vi "Actor Core_Temp.vi"() -> ()   [LabVIEW 2023, in "SLM_Controller.lvlib" / "SLM_Controller.lvclass"]
uses:
  SLM_Controller.lvclass
  SLM_Controller.lvclass/SLM_Controller.ctl
panel:
  out "Background Zero Array":i8[][](array[numeric])
  out "Background  Graph":sgl[][](graph)
  out "Background Phases":dbl[][][](array[numeric])
  out "Aperture Mask":sgl[][](array[numeric])
  out "Python session 2":refnum<k35>
  out "Python session 1":refnum<k35>
  out "SLM Max Width":i32
  out "SLM Max Height":i32
  out "slm error out 2":errorcluster
  out "Zero array":i8[][](array[numeric])
  out "Control File Path":path
  out "Phases":dbl[][][](array[numeric])
  in  "SLM Width":i32=600
  in  "SLM Height":i32=600
  out "Current Phases":sgl[][](graph)
  in  "SLM Phases":T1(tab)
  in  "Grating Sliders":T2 {"Y" scale=0.0..50.0; "X" scale=0.0..50.0}
  in  "SuperPixel Y":i8=1 min=1
  in  "SuperPixel X":i8=1 min=1
  in  "SuperPixel Array":sgl[][](array[numeric]) min=0 max=2 format="%#_3g"
  in  "SuperPixelArray_On_Off":bool
  in  "Checkerboard":T3={"Multiplier A"=0.0, "Multiplier B"=0.0, "Super Pixel Y"=1, "Super Pixel X"=1} {"Super Pixel X" min=1; "Super Pixel Y" min=1; "Multiplier B" scale=0.0..2.0; "Multiplier A" scale=0.0..2.0}
  in  "Phase Array Checkerboard":bool
  in  "Fresnel_On_Off":bool
  in  "Fresnel Lens":T4={"Wavelength"=1, "Focal Length"=1.0, "N"=0.0, "x_0"=0.0, "y_0"=0.0} {"y_0" scale=0.0..100.0; "x_0" scale=0.0..100.0; "N" scale=1.0..10.0; "Focal Length" min=1.0 max=500.0 scale=1.0..2000.0; "Wavelength" min=1 scale=1.0..1000.0}
  in  "Vortex Checkerboard On/Off":bool
  in  "Vortex_On_Off":bool
  in  "Vortex Checkerboard":T5={"Topological Charge A"=0, "Topological Charge B"=0, "VortexPixel Y"=1, "VortexPixel X"=1} {"VortexPixel X" min=1; "VortexPixel Y" min=1; "Topological Charge B" scale=-10.0..10.0; "Topological Charge A" scale=-10.0..10.0}
  in  "VortexPixel X":i8=1 min=1
  in  "VortexPixel Y":i8=1 min=1
  in  "Vortex Array":dbl[][](array[numeric])
  in  "Laguerre_On_Off":bool
  in  "Laguerre_Gaussian":T6={"L"=1, "P"=0, "w_0"=1, "x_0"=0.0, "y_0"=0.0} {"y_0" scale=0.0..100.0; "x_0" scale=0.0..100.0; "w_0" min=1 max=500 scale=1.0..500.0; "P" min=0 step=1 scale=0.0..10.0; "L" min=1 scale=1.0..10.0}
  in  "Hermite Gaussian":T7={"n"=1, "m"=0, "w_0"=1.0, "x_0"=0.0, "y_0"=0.0} {"y_0" scale=0.0..100.0; "x_0" scale=0.0..100.0; "w_0" min=1.0 max=500.0 scale=1.0..500.0; "m" min=0 step=1 scale=0.0..10.0; "n" min=1 scale=1.0..10.0}
  in  "Hermite_On_Off":bool
  in  "Axicon_On_Off":bool
  in  "Axicon Settings":cluster{"r_0":dbl, "x_0":dbl, "y_0":dbl}={"r_0"=1.0, "x_0"=0.0, "y_0"=0.0} {"y_0" scale=0.0..100.0; "x_0" scale=0.0..100.0; "r_0" min=1.0 scale=1.0..100.0}
  in  "Bessel_On_Off":bool
  in  "Bessel Settings":T8={"Topological Charge"=1, "Wavelength"=1, "Refractive Index"=0.0, "Degree"=0.0} {"Degree" scale=0.0..2.0; "Refractive Index" scale=0.0..2.0; "Wavelength" min=1 scale=1.0..1000.0; "Topological Charge" min=1 scale=1.0..10.0}
  in  "Airy_On_Off":bool
  in  "Airy Settings":cluster{"Power":i8, "Denominator":i8} {"Denominator" scale=1.0..10.0; "Power" scale=0.0..10.0}
  in  "Options Tap":enum32{"Aperture", "Background"}(tab)
  in  "Aperture Array":i16[][](array[numeric]) min=1
  in  "Aperture Pixel Y":i8=1 min=1
  in  "Aperture Pixel X":i8=1 min=1
  in  "Aperture Checkerboard":T9={"Multiplier A"=1, "Multiplier B"=1, "Aperture Pixel Y"=1, "Aperture Pixel X"=1} {"Aperture Pixel X" min=1; "Aperture Pixel Y" min=1; "Multiplier B" min=1 scale=1.0..500.0; "Multiplier A" min=1 scale=1.0..800.0}
  in  "Aperture Checkerboard On/Off":bool
  in  "Background_Axicon_On_Off":bool
  in  "Background_Grating_On_Off":bool
  in  "Background_Fresnel_On_Off":bool
  in  "Fresnel":T4={"Wavelength"=1, "Focal Length"=1.0, "N"=0.0, "x_0"=0.0, "y_0"=0.0} {"Focal Length" min=1.0 max=500.0; "Wavelength" min=1}
  in  "Grating":T2
  in  "Axicon":cluster{"r_0":dbl, "x_0":dbl, "y_0":dbl}={"r_0"=1.0, "x_0"=0.0, "y_0"=0.0} {"r_0" min=1.0}
  out "Final Phase":dbl[][](graph)
  out "phases error out":errorcluster
  in  "Modulation Depth":dbl=214.0
  in  "SLM Monitor":i32=2
  in  "Correction Pattern":path=path "C:/Users/quantum/Desktop/SLM_SImple_GUI/correction_pattern_13138/CAL_LSH0802650_810nm.bmp"
  in  "Initialize SLM":bool
  in  "Continuous Button":bool
  in  "Single Upload":bool
  in  "Start/Stop":bool
  # "X"
  # "Y"
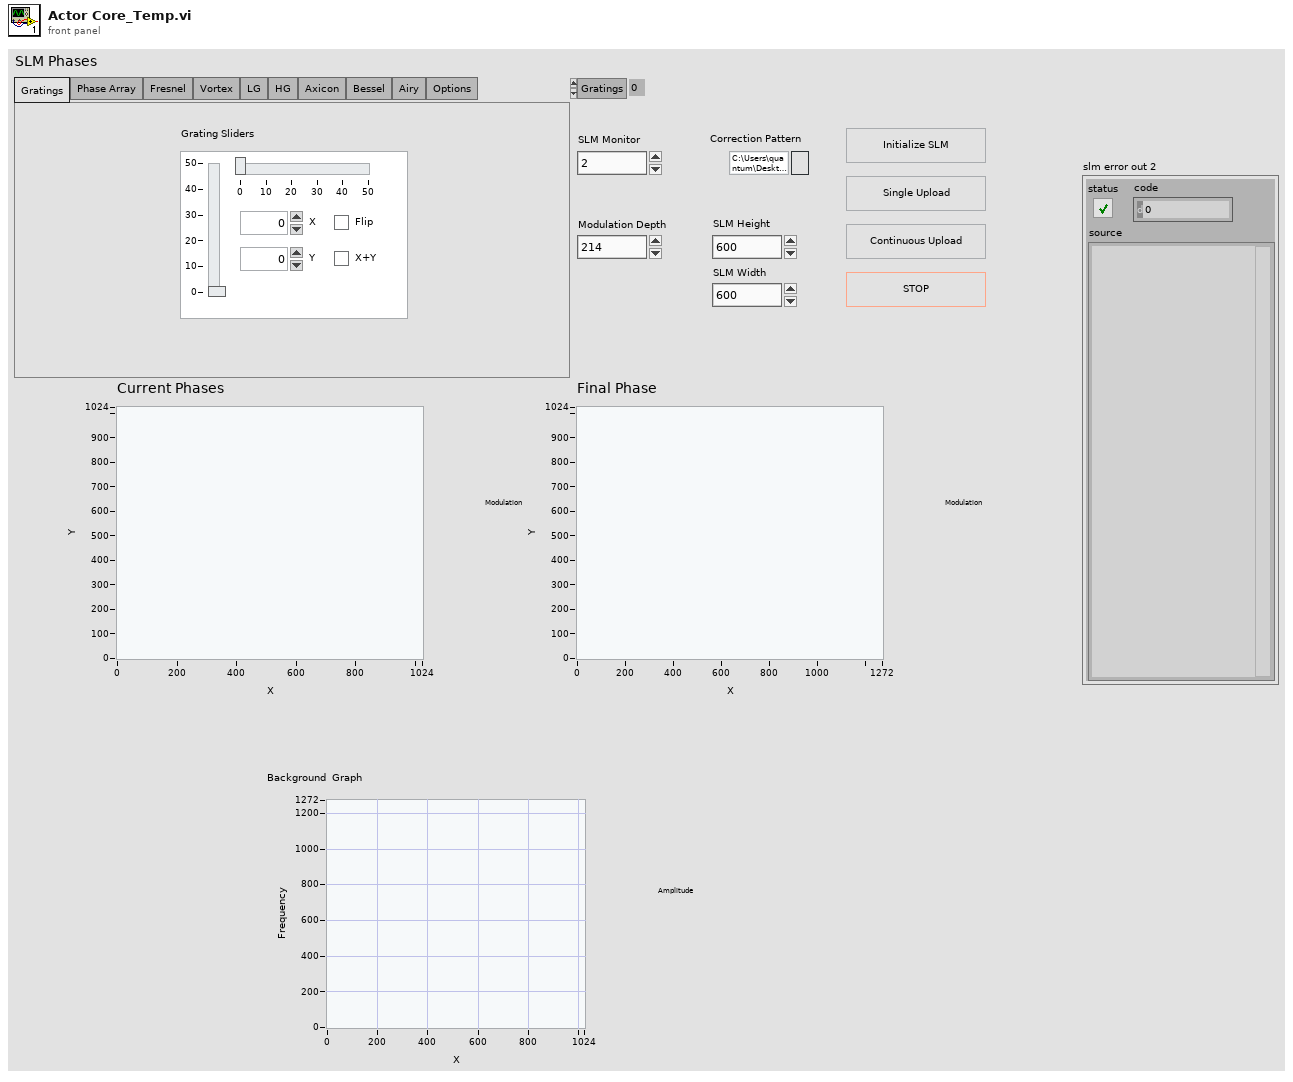
[diagram p1: front panel]
types:
  T1 = enum32{"Gratings", "Phase Array", "Fresnel", "Vortex", "LG", "HG", "Axicon", "Bessel", "Airy", "Options"}
  T2 = cluster{"X":i16, "Y":i16, "Flip":bool, "Orientation":bool}
  T3 = cluster{"Multiplier A":sgl, "Multiplier B":sgl, "Super Pixel Y":i8, "Super Pixel X":i8}
  T4 = cluster{"Wavelength":i16, "Focal Length":dbl, "N":dbl, "x_0":dbl, "y_0":dbl}
  T5 = cluster{"Topological Charge A":i8, "Topological Charge B":i8, "VortexPixel Y":i8, "VortexPixel X":i8}
  T6 = cluster{"L":i8, "P":i8, "w_0":i16, "x_0":dbl, "y_0":dbl}
  T7 = cluster{"n":i8, "m":i8, "w_0":dbl, "x_0":dbl, "y_0":dbl}
  T8 = cluster{"Topological Charge":i8, "Wavelength":i16, "Refractive Index":sgl, "Degree":sgl}
  T9 = cluster{"Multiplier A":i16, "Multiplier B":i16, "Aperture Pixel Y":i8, "Aperture Pixel X":i8}
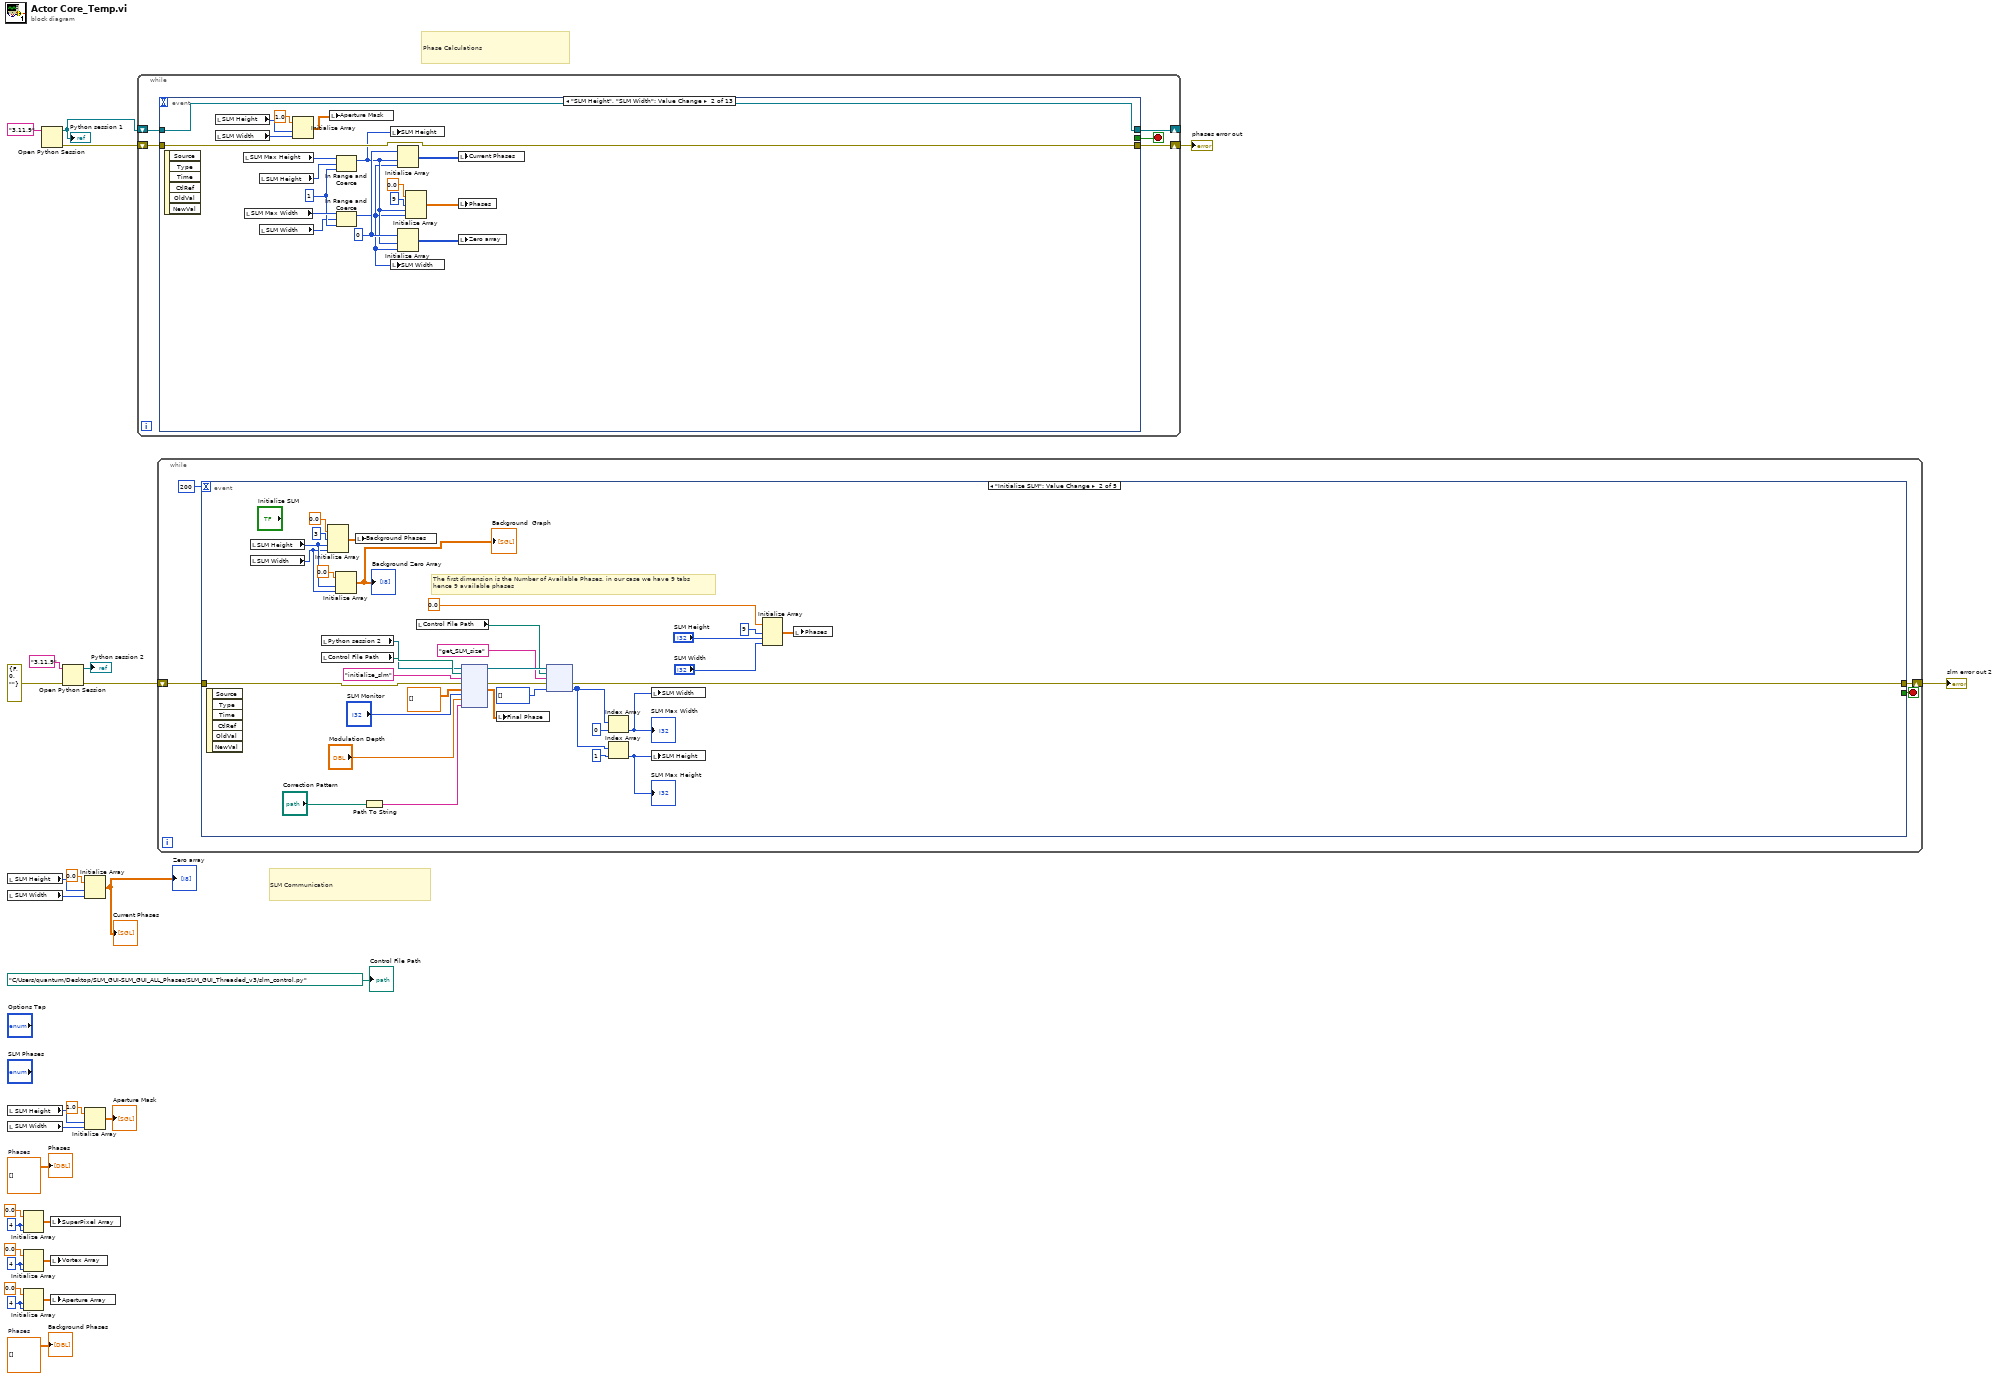
[diagram p0: block diagram]
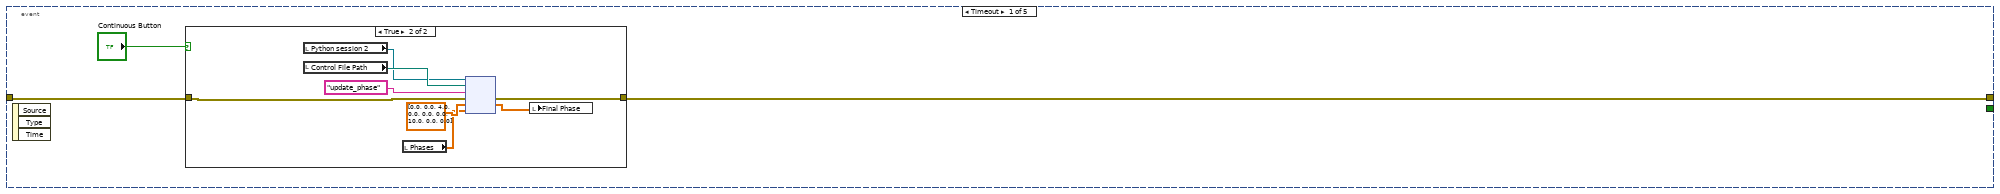
[diagram p2: hidden frame]
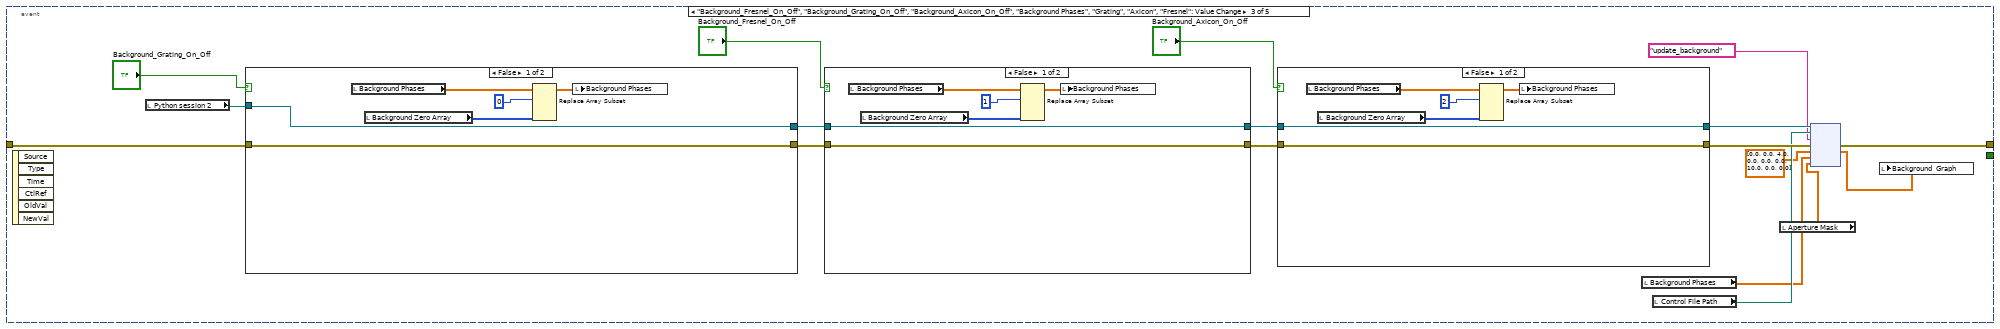
[diagram p4: hidden frame]
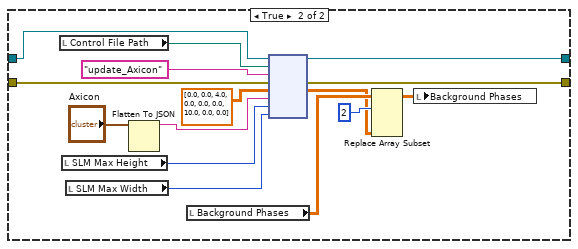
[diagram p5: hidden frame]
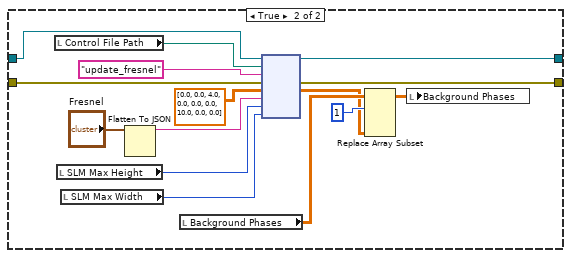
[diagram p6: hidden frame]
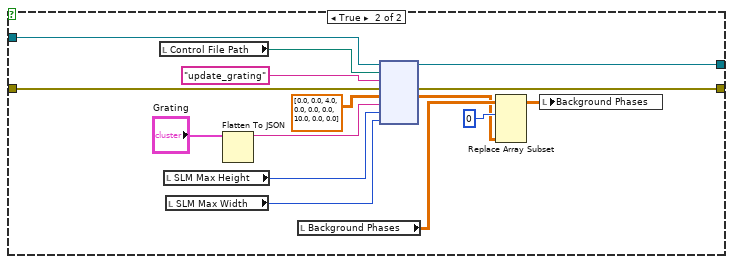
[diagram p7: hidden frame]
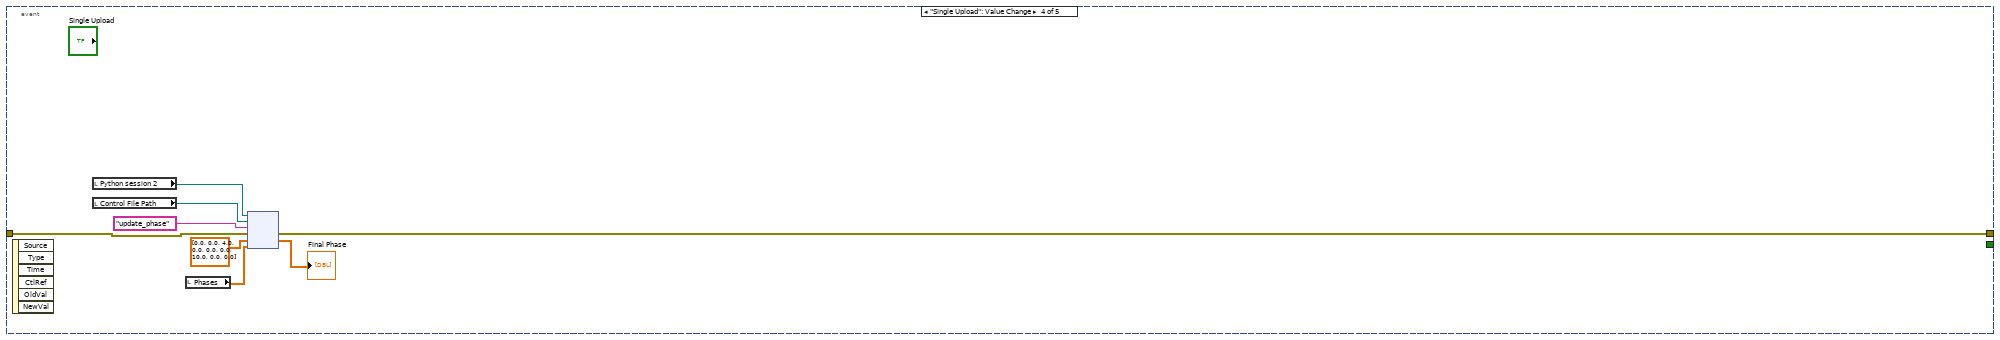
[diagram p8: hidden frame]
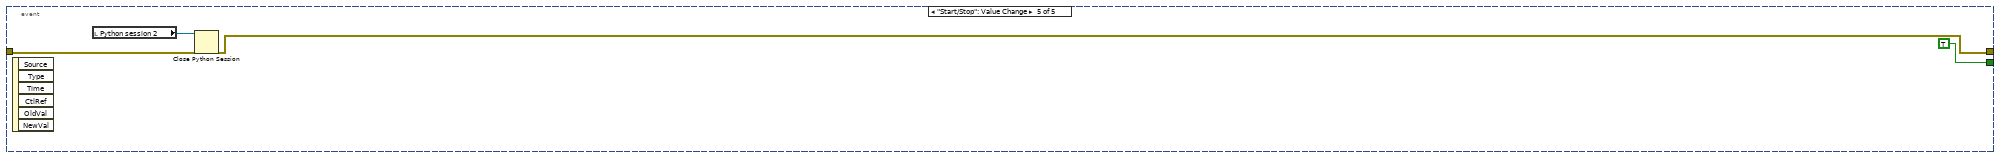
[diagram p9: hidden frame]
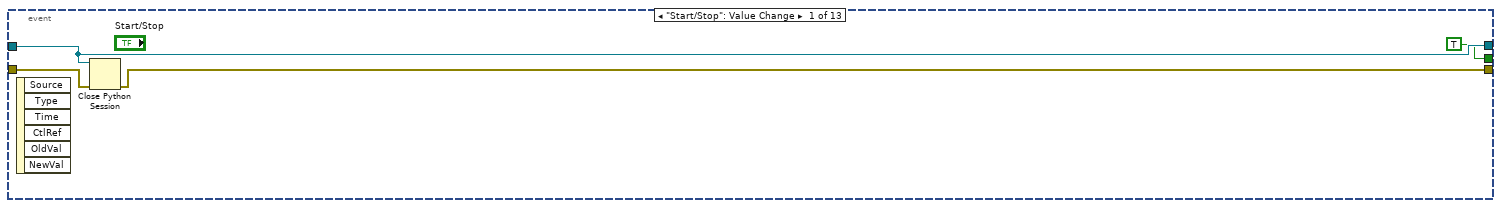
[diagram p10: hidden frame]
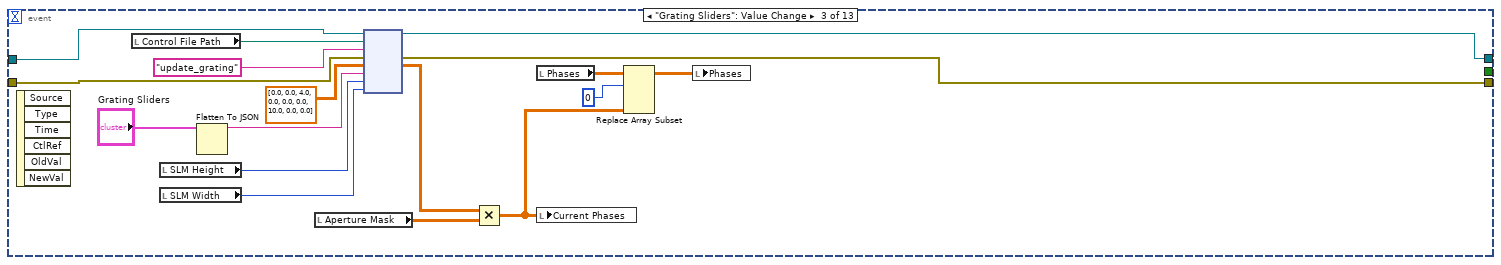
[diagram p11: hidden frame]
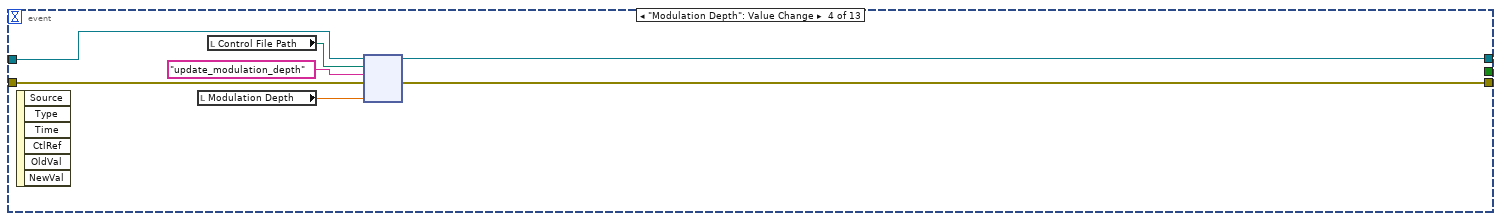
[diagram p12: hidden frame]
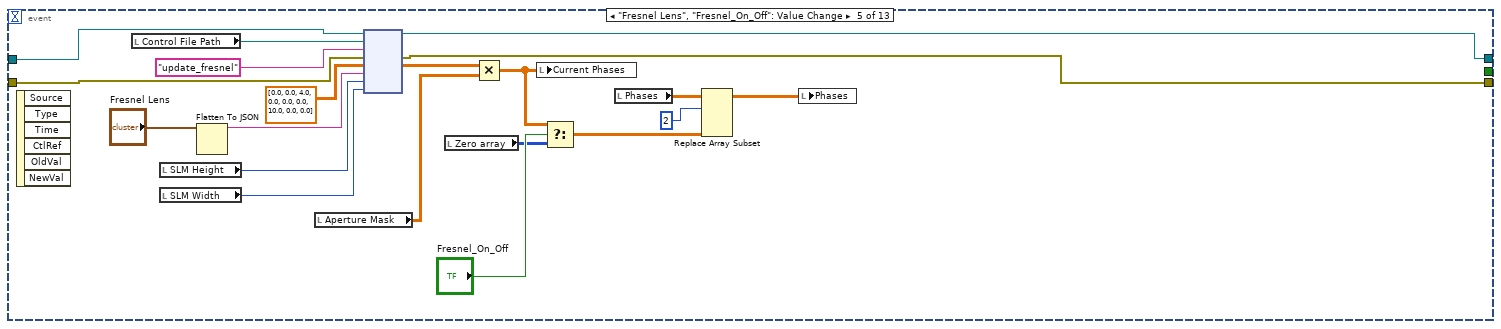
[diagram p13: hidden frame]
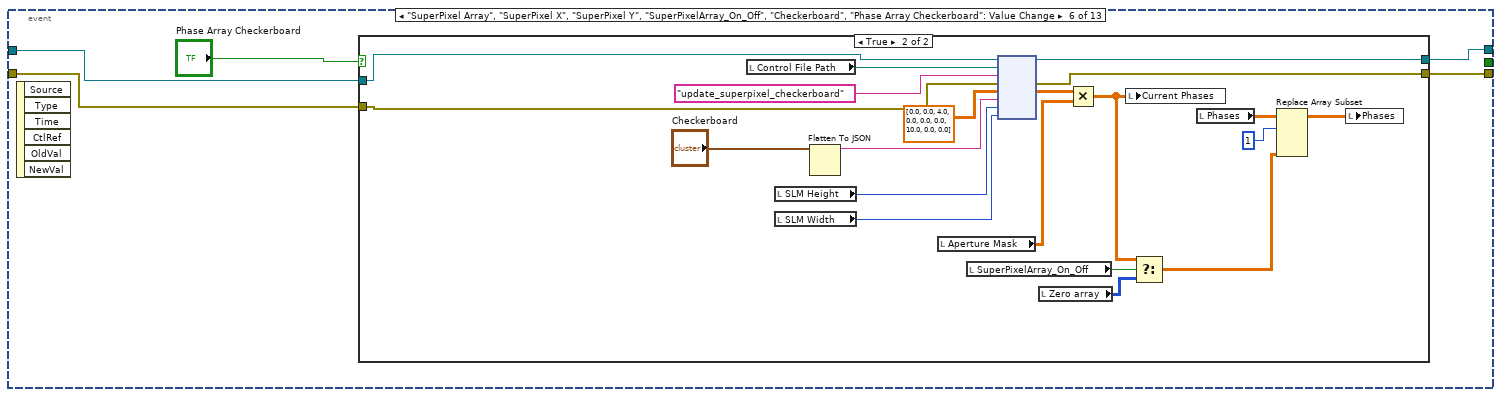
[diagram p14: hidden frame]
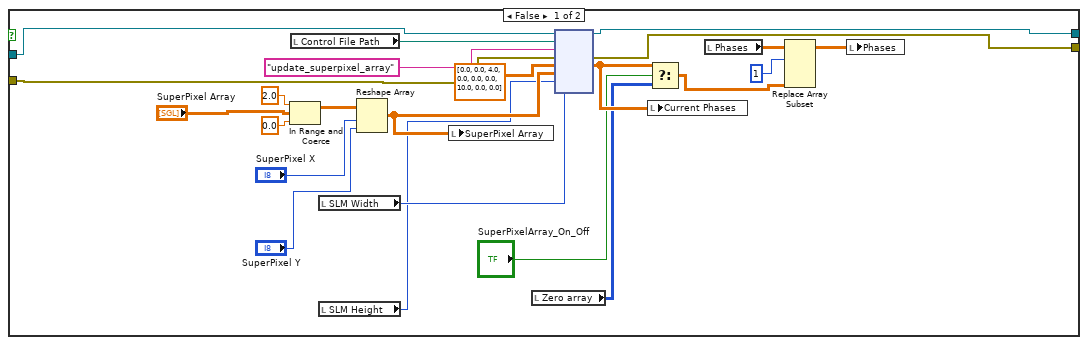
[diagram p15: hidden frame]
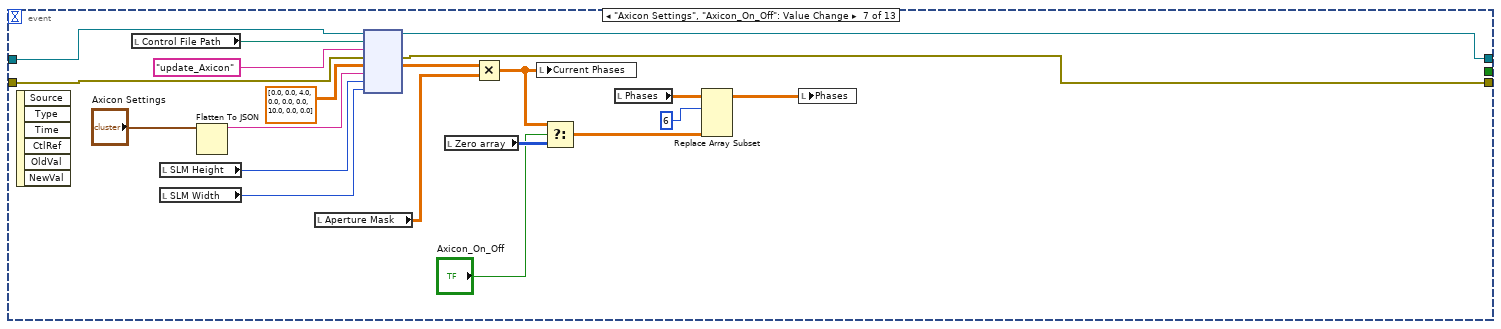
[diagram p16: hidden frame]
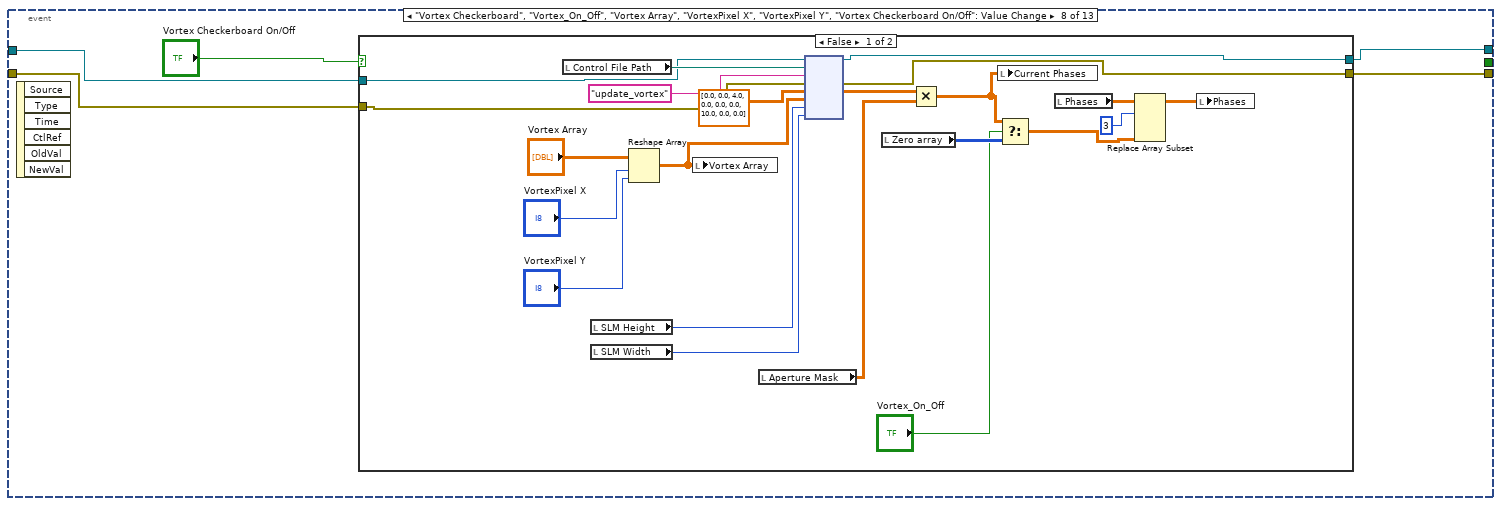
[diagram p17: hidden frame]
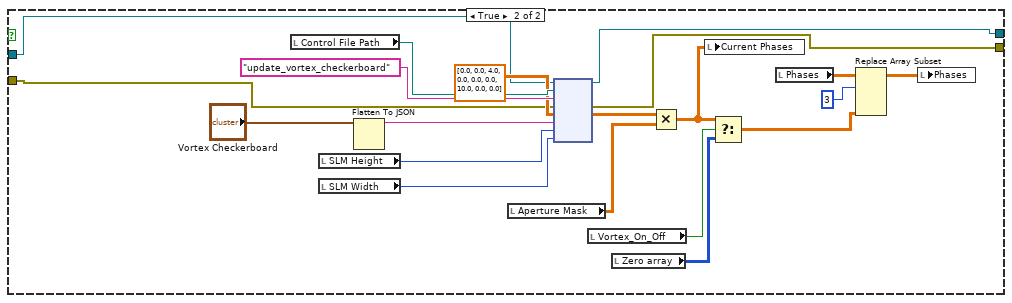
[diagram p18: hidden frame]
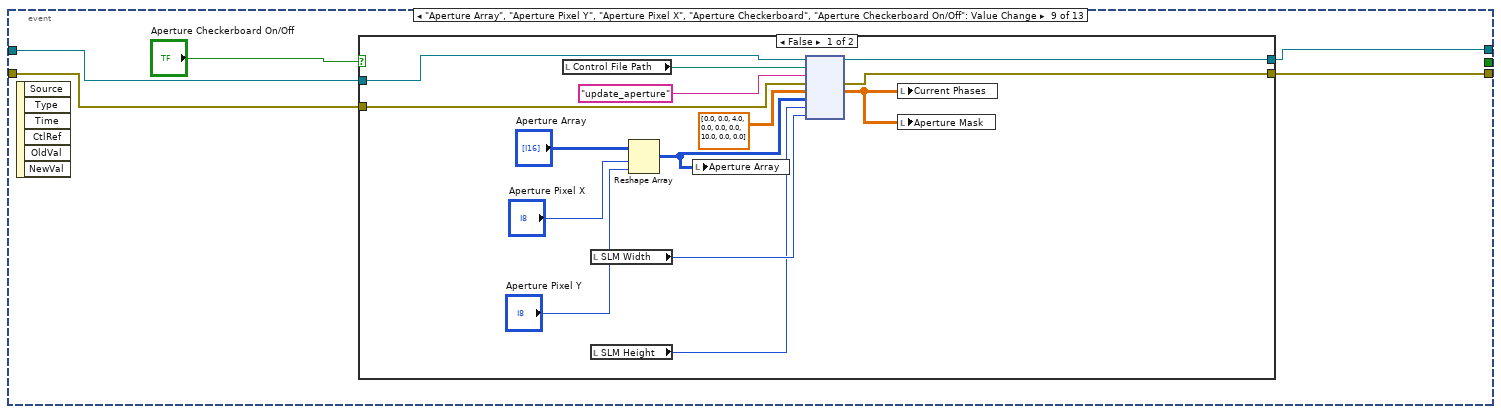
[diagram p19: hidden frame]
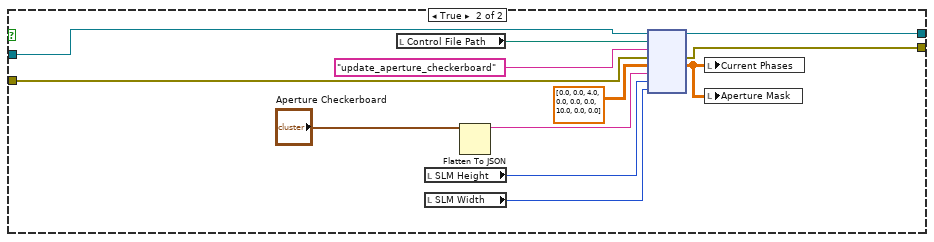
[diagram p20: hidden frame]
diagram:
  w2 = dbl[][][] []  # Phases
  w7 = 4
  w17 = 4
  w19 = 4
  w25 = dbl[][][] []  # Phases
  # "Phase Calculations"
  # "SLM Communication"
  n1 = local read "SLM Height"() -> (w23:i32)
  n2 = local read "SLM Width"() -> (w24:i32)
  n3 = local read "SLM Height"() -> (w5:i32)
  n4 = local read "SLM Width"() -> (w4:i32)
  n5 = Initialize Array(0.0 ("element"), w19, w19) -> (w16:dbl[][])
  n6 = Initialize Array(0.0 ("element"), w17, w17) -> (w15:dbl[][])
  n7 = Initialize Array(0.0 ("element"), w7, w7) -> (w9:dbl[][])
  n8 = Open Python Session(python version="3.11.9" ("Python version")) -> (session out=w29:refnum<k35>, error out=w28:errorcluster)  [unwired: 2 in]
  "Python session 1" <- w29
  n9 = local write "SuperPixel Array"(w16) -> ()
  n10 = local write "Vortex Array"(w15) -> ()
  n11 = local write "Aperture Array"(w9) -> ()
  n12 = Open Python Session(python version="3.11.9" ("Python version"), 3:errorcluster {"status"=FALSE, "code"=0, "source"=""} ("error in (no error)")) -> (session out=→"Python session 2":refnum<k35>, error out=w13:errorcluster)  [unwired: 1 in]
  n13 = Initialize Array(sgl 0.0, w23, w24) -> (→"Current Phases" →"Zero array":sgl[][])
  n14 = Initialize Array(sgl 1.0 ("element"), w5, w4) -> (→"Aperture Mask":sgl[][])
  n15 = while {
    shift-right: [w30] -> _
    shift-left: w29 -> [w34]
    shift-right: [w31] -> w26
    shift-left: w28 -> [w33]
    stop <- w32 stop-if-true
    n16 = event shown="[1] \"SLM Height\", \"SLM Width\": Value Change" {
      selector: _ -> [_ _ _ _ _ _ _ _ _ _ _ _ _]
      dyn-events: _ -> [_ _ _ _ _ _ _ _ _ _ _ _ _]
      timeout: _ -> [_ _ _ _ _ _ _ _ _ _ _ _ _]
      tunnel: w34 -> [w36 w57 w74 w80 w101 w104 w169 w174 w221 w267 w287 w307 w327]
      tunnel: w33 -> [w38 w56 w73 w79 w100 w103 w168 w172 w219 w266 w286 w306 w326]
      tunnel: [w37 w56 w61 w75 w85 w105 w153 w171 w218 w251 w271 w291 w311] -> w31
      tunnel: [w36 w57 w62 w76 w86 w106 w154 w173 w220 w252 w272 w292 w312] -> w30
      tunnel: [TRUE ("Start/Stop") _ _ _ _ _ _ _ _ _ _ _ _] -> w32
      event "Start/Stop": Value Change {
        n17 = event-data() -> ()  [unwired: 1 in, 6 out]
        n18 = Close Python Session(session in=w36, error in=w38) -> (11:w37:errorcluster)
      }
      event "SLM Height", "SLM Width": Value Change {
        w47 = 1
        w51 = 0
        n19 = event-data() -> ()  [unwired: 1 in, 6 out]
        n20 = local read "SLM Height"() -> (w41:i32)
        n21 = local read "SLM Width"() -> (w40:i32)
        n22 = local read "SLM Max Height"() -> (w49:i32)
        n23 = local read "SLM Max Width"() -> (w48:i32)
        n24 = local read "SLM Height"() -> (w46:i32)
        n25 = local read "SLM Width"() -> (w45:i32)
        n26 = Initialize Array(sgl 1.0 ("element"), w41, w40) -> (w42:sgl[][])
        n27 = local write "Aperture Mask"(w42) -> ()
        n28 = In Range and Coerce(upper limit=w49, x=w46, lower limit=w47) -> (coerced(x)=w44:i32)  [unwired: 1 out]
        n29 = In Range and Coerce(upper limit=w48, x=w45, lower limit=w47) -> (coerced(x)=w43:i32)  [unwired: 1 out]
        n30 = local write "SLM Height"(w44) -> ()
        n31 = local write "SLM Width"(w43) -> ()
        n32 = Initialize Array(w51, w44, w43) -> (w53:i32[][])
        n33 = Initialize Array(w51, w44, w43) -> (w50:i32[][])
        n34 = Initialize Array(0.0, 9, w44, w43) -> (w54:dbl[][][])
        n35 = local write "Current Phases"(w53) -> ()
        n36 = local write "Phases"(w54) -> ()
        n37 = local write "Zero array"(w50) -> ()
      }
      event "Grating Sliders": Value Change {
        n38 = event-data() -> ()  [unwired: 1 in, 6 out]
        n39 = local read "Control File Path"() -> (w72:path)
        n40 = local read "SLM Height"() -> (w67:i32)
        n41 = local read "SLM Width"() -> (w66:i32)
        n42 = Flatten To JSON(anything="Grating Sliders") -> (JSON string=w69:string)  [unwired: 2 in, 1 out]
        n43 = local read "Aperture Mask"() -> (w59:sgl[][])
        n44 = node(w74, w72, "update_grating" ("function name"), w73, dbl[][] [[0.0, 0.0, 4.0], [0.0, 0.0, 0.0], [10.0, 0.0, 0.0]] ("Python Graph"), w69, w67, w66) -> (w62:refnum<k35>, w61:errorcluster, w60:dbl[][])  [unwired: 3 in, 2 out]
        n45 = Multiply(x=w60, y=w59) -> (x*y=w58:dbl[][])
        n46 = local read "Phases"() -> (w65:dbl[][][])
        n47 = local write "Current Phases"(w58) -> ()
        n48 = Replace Array Subset(array=w65, new element=w58, index (dim 0)=0 ("index (page)")) -> (w64:dbl[][][])  [unwired: 2 in]
        n49 = local write "Phases"(w64) -> ()
      }
      event "Modulation Depth": Value Change {
        n50 = event-data() -> ()  [unwired: 1 in, 6 out]
        n51 = local read "Modulation Depth"() -> (w78:dbl)
        n52 = local read "Control File Path"() -> (w81:path)
        n53 = node(w80, w81, "update_modulation_depth" ("function name"), w79, w78) -> (w76:refnum<k35>, w75:errorcluster)  [unwired: 3 in, 2 out]
      }
      event "Fresnel Lens", "Fresnel_On_Off": Value Change {
        n54 = event-data() -> ()  [unwired: 1 in, 6 out]
        n55 = local read "Control File Path"() -> (w96:path)
        n56 = local read "SLM Height"() -> (w94:i32)
        n57 = local read "SLM Width"() -> (w93:i32)
        n58 = Flatten To JSON(anything="Fresnel Lens") -> (JSON string=w97:string)  [unwired: 2 in, 1 out]
        n59 = local read "Aperture Mask"() -> (w83:sgl[][])
        n60 = node(w101, w96, "update_fresnel" ("function name"), w100, dbl[][] [[0.0, 0.0, 4.0], [0.0, 0.0, 0.0], [10.0, 0.0, 0.0]] ("Python Graph"), w97, w94, w93) -> (w86:refnum<k35>, w85:errorcluster, w84:dbl[][])  [unwired: 3 in, 2 out]
        n61 = local read "Zero array"() -> (w88:i8[][])
        n62 = Multiply(x=w84, y=w83) -> (x*y=w82:dbl[][])
        n63 = local write "Current Phases"(w82) -> ()
        n64 = Select(t=w82, s="Fresnel_On_Off", f=w88) -> (s? t:f=w87:dbl[][])
        n65 = local read "Phases"() -> (w92:dbl[][][])
        n66 = Replace Array Subset(array=w92, new element=w87, index (dim 0)=2 ("index (page)")) -> (w91:dbl[][][])  [unwired: 2 in]
        n67 = local write "Phases"(w91) -> ()
      }
      event "SuperPixel Array", "SuperPixel X", "SuperPixel Y", "SuperPixelArray_On_Off", "Checkerboard", "Phase Array Checkerboard": Value Change {
        n68 = event-data() -> ()  [unwired: 1 in, 6 out]
        n69 = case shown="True" "Phase Array Checkerboard" {
          tunnel: [w110 w136] -> w106
          tunnel: [w109 w135] -> w105
          tunnel: w104 -> [w108 w138]
          tunnel: w103 -> [w107 w137]
          frame False {
            n70 = In Range and Coerce(upper limit=2.0, x="SuperPixel Array", lower limit=0.0) -> (coerced(x)=w122:dbl[][])  [unwired: 1 out]
            n71 = local read "Control File Path"() -> (w116:path)
            n72 = local read "SLM Width"() -> (w118:i32)
            n73 = local read "SLM Height"() -> (w117:i32)
            n74 = Reshape Array(w122, "SuperPixel X", "SuperPixel Y") -> (w123:dbl[][])
            n75 = local write "SuperPixel Array"(w123) -> ()
            n76 = local read "Zero array"() -> (w126:i8[][])
            n77 = node(w108, w116, "update_superpixel_array" ("function name"), w107, dbl[][] [[0.0, 0.0, 4.0], [0.0, 0.0, 0.0], [10.0, 0.0, 0.0]] ("Python Graph"), w123, w117, w118) -> (w110:refnum<k35>, w109:errorcluster, w128:dbl[][])  [unwired: 3 in, 2 out]
            n78 = local write "Current Phases"(w128) -> ()
            n79 = Select(t=w128, s="SuperPixelArray_On_Off", f=w126) -> (s? t:f=w129:dbl[][])
            n80 = local read "Phases"() -> (w124:dbl[][][])
            n81 = Replace Array Subset(array=w124, new element=w129, index (dim 0)=1) -> (w125:dbl[][][])  [unwired: 2 in]
            n82 = local write "Phases"(w125) -> ()
          }
          frame True {
            n83 = local read "Control File Path"() -> (w143:path)
            n84 = local read "SLM Height"() -> (w144:i32)
            n85 = local read "SLM Width"() -> (w145:i32)
            n86 = Flatten To JSON(anything="Checkerboard") -> (JSON string=w133:string)  [unwired: 2 in, 1 out]
            n87 = local read "Aperture Mask"() -> (w131:sgl[][])
            n88 = local read "SuperPixelArray_On_Off"() -> (w139:bool)
            n89 = node(w138, w143, "update_superpixel_checkerboard" ("function name"), w137, dbl[][] [[0.0, 0.0, 4.0], [0.0, 0.0, 0.0], [10.0, 0.0, 0.0]] ("Python Graph"), w133, w144, w145) -> (w136:refnum<k35>, w135:errorcluster, w132:dbl[][])  [unwired: 3 in, 2 out]
            n90 = local read "Zero array"() -> (w148:i8[][])
            n91 = Multiply(x=w132, y=w131) -> (x*y=w130:dbl[][])
            n92 = local write "Current Phases"(w130) -> ()
            n93 = Select(t=w130, s=w139, f=w148) -> (s? t:f=w149:dbl[][])
            n94 = local read "Phases"() -> (w146:dbl[][][])
            n95 = Replace Array Subset(array=w146, new element=w149, index (dim 0)=1) -> (w147:dbl[][][])  [unwired: 2 in]
            n96 = local write "Phases"(w147) -> ()
          }
        }
      }
      event "Axicon Settings", "Axicon_On_Off": Value Change {
        n97 = event-data() -> ()  [unwired: 1 in, 6 out]
        n98 = local read "Control File Path"() -> (w165:path)
        n99 = local read "SLM Height"() -> (w162:i32)
        n100 = local read "SLM Width"() -> (w161:i32)
        n101 = Flatten To JSON(anything="Axicon Settings") -> (JSON string=w166:string)  [unwired: 2 in, 1 out]
        n102 = local read "Aperture Mask"() -> (w151:sgl[][])
        n103 = node(w169, w165, "update_Axicon" ("function name"), w168, dbl[][] [[0.0, 0.0, 4.0], [0.0, 0.0, 0.0], [10.0, 0.0, 0.0]] ("Python Graph"), w166, w162, w161) -> (w154:refnum<k35>, w153:errorcluster, w152:dbl[][])  [unwired: 3 in, 2 out]
        n104 = local read "Zero array"() -> (w157:i8[][])
        n105 = Multiply(x=w152, y=w151) -> (x*y=w150:dbl[][])
        n106 = local write "Current Phases"(w150) -> ()
        n107 = Select(t=w150, s="Axicon_On_Off", f=w157) -> (s? t:f=w155:dbl[][])
        n108 = local read "Phases"() -> (w159:dbl[][][])
        n109 = Replace Array Subset(array=w159, new element=w155, index (dim 0)=6 ("index (page)")) -> (w160:dbl[][][])  [unwired: 2 in]
        n110 = local write "Phases"(w160) -> ()
      }
      event "Vortex Checkerboard", "Vortex_On_Off", "Vortex Array", "VortexPixel X", "VortexPixel Y", "Vortex Checkerboard On/Off": Value Change {
        n111 = event-data() -> ()  [unwired: 1 in, 6 out]
        n112 = case shown="False" "Vortex Checkerboard On/Off" {
          tunnel: w174 -> [w183 w206]
          tunnel: [w180 w204] -> w173
          tunnel: w172 -> [w179 w205]
          tunnel: [w178 w203] -> w171
          frame False {
            n113 = local read "Control File Path"() -> (w185:path)
            n114 = local read "SLM Height"() -> (w186:i32)
            n115 = local read "SLM Width"() -> (w187:i32)
            n116 = Reshape Array("Vortex Array", "VortexPixel X", "VortexPixel Y") -> (w196:dbl[][])
            n117 = local write "Vortex Array"(w196) -> ()
            n118 = local read "Aperture Mask"() -> (w176:sgl[][])
            n119 = node(w183, w185, "update_vortex" ("function name"), w179, dbl[][] [[0.0, 0.0, 4.0], [0.0, 0.0, 0.0], [10.0, 0.0, 0.0]] ("Python Graph"), w196, w186, w187) -> (w180:refnum<k35>, w178:errorcluster, w177:dbl[][])  [unwired: 3 in, 2 out]
            n120 = local read "Zero array"() -> (w191:i8[][])
            n121 = Multiply(x=w177, y=w176) -> (x*y=w175:dbl[][])
            n122 = local write "Current Phases"(w175) -> ()
            n123 = Select(t=w175, s="Vortex_On_Off", f=w191) -> (s? t:f=w192:dbl[][])
            n124 = local read "Phases"() -> (w189:dbl[][][])
            n125 = Replace Array Subset(array=w189, new element=w192, index (dim 0)=3 ("index (page)")) -> (w188:dbl[][][])  [unwired: 2 in]
            n126 = local write "Phases"(w188) -> ()
          }
          frame True {
            n127 = local read "Control File Path"() -> (w210:path)
            n128 = local read "SLM Height"() -> (w211:i32)
            n129 = local read "SLM Width"() -> (w212:i32)
            n130 = Flatten To JSON(anything="Vortex Checkerboard") -> (JSON string=w200:string)  [unwired: 2 in, 1 out]
            n131 = local read "Aperture Mask"() -> (w198:sgl[][])
            n132 = node(w206, w210, "update_vortex_checkerboard" ("function name"), w205, dbl[][] [[0.0, 0.0, 4.0], [0.0, 0.0, 0.0], [10.0, 0.0, 0.0]] ("Python Graph"), w200, w211, w212) -> (w204:refnum<k35>, w203:errorcluster, w199:dbl[][])  [unwired: 3 in, 2 out]
            n133 = local read "Vortex_On_Off"() -> (w202:bool)
            n134 = local read "Zero array"() -> (w215:i8[][])
            n135 = Multiply(x=w199, y=w198) -> (x*y=w197:dbl[][])
            n136 = local write "Current Phases"(w197) -> ()
            n137 = Select(t=w197, s=w202, f=w215) -> (s? t:f=w216:dbl[][])
            n138 = local read "Phases"() -> (w214:dbl[][][])
            n139 = Replace Array Subset(array=w214, new element=w216, index (dim 0)=3 ("index (page)")) -> (w213:dbl[][][])  [unwired: 2 in]
            n140 = local write "Phases"(w213) -> ()
          }
        }
      }
      event "Aperture Array", "Aperture Pixel Y", "Aperture Pixel X", "Aperture Checkerboard", "Aperture Checkerboard On/Off": Value Change {
        n141 = event-data() -> ()  [unwired: 1 in, 6 out]
        n142 = case shown="False" "Aperture Checkerboard On/Off" {
          tunnel: w221 -> [w231 w242]
          tunnel: [w228 w240] -> w220
          tunnel: w219 -> [w227 w241]
          tunnel: [w226 w239] -> w218
          frame False {
            n143 = local read "Control File Path"() -> (w232:path)
            n144 = local read "SLM Width"() -> (w234:i32)
            n145 = local read "SLM Height"() -> (w233:i32)
            n146 = Reshape Array("Aperture Array", "Aperture Pixel X", "Aperture Pixel Y") -> (w235:i16[][])
            n147 = local write "Aperture Array"(w235) -> ()
            n148 = node(w231, w232, "update_aperture" ("function name"), w227, dbl[][] [[0.0, 0.0, 4.0], [0.0, 0.0, 0.0], [10.0, 0.0, 0.0]] ("Python Graph"), w235, w233, w234) -> (w228:refnum<k35>, w226:errorcluster, w222:dbl[][])  [unwired: 3 in, 2 out]
            n149 = local write "Current Phases"(w222) -> ()
            n150 = local write "Aperture Mask"(w222) -> ()
          }
          frame True {
            n151 = local read "Control File Path"() -> (w245:path)
            n152 = local read "SLM Height"() -> (w246:i32)
            n153 = local read "SLM Width"() -> (w247:i32)
            n154 = Flatten To JSON(anything="Aperture Checkerboard") -> (JSON string=w238:string)  [unwired: 2 in, 1 out]
            n155 = node(w242, w245, "update_aperture_checkerboard" ("function name"), w241, dbl[][] [[0.0, 0.0, 4.0], [0.0, 0.0, 0.0], [10.0, 0.0, 0.0]] ("Python Graph"), w238, w246, w247) -> (w240:refnum<k35>, w239:errorcluster, w236:dbl[][])  [unwired: 3 in, 2 out]
            n156 = local write "Current Phases"(w236) -> ()
            n157 = local write "Aperture Mask"(w236) -> ()
          }
        }
      }
      event "Laguerre_Gaussian", "Laguerre_On_Off": Value Change {
        n158 = event-data() -> ()  [unwired: 1 in, 6 out]
        n159 = local read "Control File Path"() -> (w263:path)
        n160 = local read "SLM Height"() -> (w260:i32)
        n161 = local read "SLM Width"() -> (w259:i32)
        n162 = Flatten To JSON(anything="Laguerre_Gaussian") -> (JSON string=w264:string)  [unwired: 2 in, 1 out]
        n163 = local read "Aperture Mask"() -> (w249:sgl[][])
        n164 = node(w267, w263, "update_LG" ("function name"), w266, dbl[][] [[0.0, 0.0, 4.0], [0.0, 0.0, 0.0], [10.0, 0.0, 0.0]] ("Python Graph"), w264, w260, w259) -> (w252:refnum<k35>, w251:errorcluster, w250:dbl[][])  [unwired: 3 in, 2 out]
        n165 = local read "Zero array"() -> (w254:i8[][])
        n166 = Multiply(x=w250, y=w249) -> (x*y=w248:dbl[][])
        n167 = local write "Current Phases"(w248) -> ()
        n168 = Select(t=w248, s="Laguerre_On_Off", f=w254) -> (s? t:f=w253:dbl[][])
        n169 = local read "Phases"() -> (w257:dbl[][][])
        n170 = Replace Array Subset(array=w257, new element=w253, index (dim 0)=4 ("index (page)")) -> (w258:dbl[][][])  [unwired: 2 in]
        n171 = local write "Phases"(w258) -> ()
      }
      event "Airy Settings", "Airy_On_Off": Value Change {
        n172 = event-data() -> ()  [unwired: 1 in, 6 out]
        n173 = local read "Control File Path"() -> (w283:path)
        n174 = local read "SLM Height"() -> (w281:i32)
        n175 = local read "SLM Width"() -> (w280:i32)
        n176 = Flatten To JSON(anything="Airy Settings") -> (JSON string=w284:string)  [unwired: 2 in, 1 out]
        n177 = local read "Aperture Mask"() -> (w269:sgl[][])
        n178 = node(w287, w283, "update_Airy" ("function name"), w286, dbl[][] [[0.0, 0.0, 4.0], [0.0, 0.0, 0.0], [10.0, 0.0, 0.0]] ("Python Graph"), w284, w281, w280) -> (w272:refnum<k35>, w271:errorcluster, w270:dbl[][])  [unwired: 3 in, 2 out]
        n179 = local read "Zero array"() -> (w274:i8[][])
        n180 = Multiply(x=w270, y=w269) -> (x*y=w268:dbl[][])
        n181 = local write "Current Phases"(w268) -> ()
        n182 = Select(t=w268, s="Airy_On_Off", f=w274) -> (s? t:f=w273:dbl[][])
        n183 = local read "Phases"() -> (w277:dbl[][][])
        n184 = Replace Array Subset(array=w277, new element=w273, index (dim 0)=8 ("index (page)")) -> (w278:dbl[][][])  [unwired: 2 in]
        n185 = local write "Phases"(w278) -> ()
      }
      event "Bessel Settings", "Bessel_On_Off": Value Change {
        n186 = event-data() -> ()  [unwired: 1 in, 6 out]
        n187 = local read "Control File Path"() -> (w303:path)
        n188 = local read "SLM Height"() -> (w301:i32)
        n189 = local read "SLM Width"() -> (w300:i32)
        n190 = Flatten To JSON(anything="Bessel Settings") -> (JSON string=w304:string)  [unwired: 2 in, 1 out]
        n191 = local read "Aperture Mask"() -> (w289:sgl[][])
        n192 = node(w307, w303, "update_Bessel" ("function name"), w306, dbl[][] [[0.0, 0.0, 4.0], [0.0, 0.0, 0.0], [10.0, 0.0, 0.0]] ("Python Graph"), w304, w301, w300) -> (w292:refnum<k35>, w291:errorcluster, w290:dbl[][])  [unwired: 3 in, 2 out]
        n193 = local read "Zero array"() -> (w295:i8[][])
        n194 = Multiply(x=w290, y=w289) -> (x*y=w288:dbl[][])
        n195 = local write "Current Phases"(w288) -> ()
        n196 = Select(t=w288, s="Bessel_On_Off", f=w295) -> (s? t:f=w293:dbl[][])
        n197 = local read "Phases"() -> (w297:dbl[][][])
        n198 = Replace Array Subset(array=w297, new element=w293, index (dim 0)=7 ("index (page)")) -> (w298:dbl[][][])  [unwired: 2 in]
        n199 = local write "Phases"(w298) -> ()
      }
      event "Hermite Gaussian", "Hermite_On_Off": Value Change {
        n200 = event-data() -> ()  [unwired: 1 in, 6 out]
        n201 = local read "Control File Path"() -> (w323:path)
        n202 = local read "SLM Height"() -> (w321:i32)
        n203 = local read "SLM Width"() -> (w320:i32)
        n204 = Flatten To JSON(anything="Hermite Gaussian") -> (JSON string=w324:string)  [unwired: 2 in, 1 out]
        n205 = local read "Aperture Mask"() -> (w309:sgl[][])
        n206 = node(w327, w323, "update_HG" ("function name"), w326, dbl[][] [[0.0, 0.0, 4.0], [0.0, 0.0, 0.0], [10.0, 0.0, 0.0]] ("Python Graph"), w324, w321, w320) -> (w312:refnum<k35>, w311:errorcluster, w310:dbl[][])  [unwired: 3 in, 2 out]
        n207 = local read "Zero array"() -> (w315:i8[][])
        n208 = Multiply(x=w310, y=w309) -> (x*y=w308:dbl[][])
        n209 = local write "Current Phases"(w308) -> ()
        n210 = Select(t=w308, s="Hermite_On_Off", f=w315) -> (s? t:f=w313:dbl[][])
        n211 = local read "Phases"() -> (w317:dbl[][][])
        n212 = Replace Array Subset(array=w317, new element=w313, index (dim 0)=5 ("index (page)")) -> (w318:dbl[][][])  [unwired: 2 in]
        n213 = local write "Phases"(w318) -> ()
      }
    }
  }
  "phases error out" <- w26
  n214 = while {
    shift-right: [w330] -> w12
    shift-left: w13 -> [w331]
    stop <- w329 stop-if-true
    n215 = event shown="[1] \"Initialize SLM\": Value Change" {
      selector: _ -> [_ _ _ _ _]
      dyn-events: _ -> [_ _ _ _ _]
      timeout: 200 -> [_ _ _ _ _]
      tunnel: w331 -> [w334 w363 w380 w460 w467]
      tunnel: [w333 w360 w381 w459 w466] -> w330
      tunnel: [_ _ _ _ TRUE] -> w329
      event Timeout {
        n216 = event-data() -> ()  [unwired: 1 in, 3 out]
        n217 = case shown="True" "Continuous Button" {
          tunnel: [w335 w343] -> w333
          tunnel: w334 -> [w335 w337]
          frame False {
          }
          frame True {
            n218 = local read "Python session 2"() -> (w336:refnum<k35>)
            n219 = local read "Control File Path"() -> (w338:path)
            n220 = local read "Phases"() -> (w339:dbl[][][])
            n221 = node(w336, w338, "update_phase" ("function name"), w337, dbl[][] [[0.0, 0.0, 4.0], [0.0, 0.0, 0.0], [10.0, 0.0, 0.0]] ("Python Graph"), w339) -> (w343:errorcluster, w340:dbl[][])  [unwired: 1 in, 3 out]
            n222 = local write "Final Phase"(w340) -> ()
          }
        }
      }
      event "Initialize SLM": Value Change {
        # "The first dimension is the Number of Available Phases, in our case we have 9 tabs\nhence 9 available phases"
        n223 = event-data() -> ()  [unwired: 1 in, 6 out]
        n224 = local read "SLM Height"() -> (w347:i32)
        n225 = local read "SLM Width"() -> (w346:i32)
        n226 = local read "Python session 2"() -> (w353:refnum<k35>)
        n227 = local read "Control File Path"() -> (w375:path)
        n228 = Initialize Array(0.0, 3, w347, w346) -> (w348:dbl[][][])
        n229 = Initialize Array(sgl 0.0, w347, w346) -> (→"Background Zero Array" →"Background  Graph":sgl[][])
        n230 = local write "Background Phases"(w348) -> ()
        n231 = Path To String(path="Correction Pattern") -> (string=w369:string)
        n232 = local read "Control File Path"() -> (w359:path)
        n233 = node(w353, w375, "initialize_slm" ("function name"), w363, dbl[][] [], "SLM Monitor", "Modulation Depth", w369) -> (w362:refnum<k35>, w361:errorcluster, w376:dbl[][])  [unwired: 3 in, 2 out]
        n234 = local write "Final Phase"(w376) -> ()
        n235 = node(w362, w359, "get_SLM_size" ("function name"), w361, i32[] []) -> (w360:errorcluster, w356:i32[])  [unwired: 3 out]
        n236 = Index Array(array=w356, index=0) -> (element=w352:i32)
        "SLM Max Width" <- w352
        n237 = Index Array(array=w356, index=1) -> (element=w351:i32)
        "SLM Max Height" <- w351
        n238 = local write "SLM Width"(w352) -> ()
        n239 = local write "SLM Height"(w351) -> ()
        n240 = Initialize Array(0.0, 9, "SLM Height", "SLM Width") -> (w374:dbl[][][])
        n241 = local write "Phases"(w374) -> ()
      }
      event "Background_Fresnel_On_Off", "Background_Grating_On_Off", "Background_Axicon_On_Off", "Background Phases", "Grating", "Axicon", "Fresnel": Value Change {
        n242 = event-data() -> ()  [unwired: 1 in, 6 out]
        n243 = local read "Python session 2"() -> (w379:refnum<k35>)
        n244 = case shown="False" "Background_Grating_On_Off" {
          tunnel: [w437 w451] -> w384
          tunnel: [w438 w450] -> w386
          tunnel: w380 -> [w437 w444]
          tunnel: w379 -> [w438 w443]
          frame False {
            n245 = local read "Background Phases"() -> (w441:dbl[][][])
            n246 = local read "Background Zero Array"() -> (w440:i8[][])
            n247 = Replace Array Subset(array=w441, new element=w440, index (dim 0)=0 ("index (page)")) -> (w442:dbl[][][])  [unwired: 2 in]
            n248 = local write "Background Phases"(w442) -> ()
          }
          frame True {
            n249 = local read "Control File Path"() -> (w454:path)
            n250 = local read "SLM Max Height"() -> (w456:i32)
            n251 = local read "SLM Max Width"() -> (w457:i32)
            n252 = Flatten To JSON(anything="Grating") -> (JSON string=w453:string)  [unwired: 2 in, 1 out]
            n253 = local read "Background Phases"() -> (w448:dbl[][][])
            n254 = node(w443, w454, "update_grating" ("function name"), w444, dbl[][] [[0.0, 0.0, 4.0], [0.0, 0.0, 0.0], [10.0, 0.0, 0.0]] ("Python Graph"), w453, w456, w457) -> (w450:refnum<k35>, w451:errorcluster, w445:dbl[][])  [unwired: 3 in, 2 out]
            n255 = Replace Array Subset(array=w448, new element=w445, index (dim 0)=0 ("index (page)")) -> (w447:dbl[][][])  [unwired: 2 in]
            n256 = local write "Background Phases"(w447) -> ()
          }
        }
        n257 = case shown="False" "Background_Fresnel_On_Off" {
          tunnel: w384 -> [w420 w430]
          tunnel: [w420 w429] -> w385
          tunnel: w386 -> [w421 w428]
          tunnel: [w421 w427] -> w387
          frame False {
            n258 = local read "Background Phases"() -> (w418:dbl[][][])
            n259 = local read "Background Zero Array"() -> (w417:i8[][])
            n260 = Replace Array Subset(array=w418, new element=w417, index (dim 0)=1 ("index (page)")) -> (w419:dbl[][][])  [unwired: 2 in]
            n261 = local write "Background Phases"(w419) -> ()
          }
          frame True {
            n262 = local read "Control File Path"() -> (w433:path)
            n263 = local read "SLM Max Height"() -> (w435:i32)
            n264 = local read "SLM Max Width"() -> (w436:i32)
            n265 = Flatten To JSON(anything="Fresnel") -> (JSON string=w432:string)  [unwired: 2 in, 1 out]
            n266 = local read "Background Phases"() -> (w424:dbl[][][])
            n267 = node(w428, w433, "update_fresnel" ("function name"), w430, dbl[][] [[0.0, 0.0, 4.0], [0.0, 0.0, 0.0], [10.0, 0.0, 0.0]] ("Python Graph"), w432, w435, w436) -> (w427:refnum<k35>, w429:errorcluster, w422:dbl[][])  [unwired: 3 in, 2 out]
            n268 = Replace Array Subset(array=w424, new element=w422, index (dim 0)=1 ("index (page)")) -> (w425:dbl[][][])  [unwired: 2 in]
            n269 = local write "Background Phases"(w425) -> ()
          }
        }
        n270 = case shown="False" "Background_Axicon_On_Off" {
          tunnel: w385 -> [w399 w409]
          tunnel: [w399 w408] -> w393
          tunnel: w387 -> [w400 w407]
          tunnel: [w400 w406] -> w394
          frame False {
            n271 = local read "Background Phases"() -> (w397:dbl[][][])
            n272 = local read "Background Zero Array"() -> (w396:i8[][])
            n273 = Replace Array Subset(array=w397, new element=w396, index (dim 0)=2 ("index (page)")) -> (w398:dbl[][][])  [unwired: 2 in]
            n274 = local write "Background Phases"(w398) -> ()
          }
          frame True {
            n275 = local read "Control File Path"() -> (w412:path)
            n276 = local read "SLM Max Height"() -> (w414:i32)
            n277 = local read "SLM Max Width"() -> (w415:i32)
            n278 = Flatten To JSON(anything="Axicon") -> (JSON string=w411:string)  [unwired: 2 in, 1 out]
            n279 = local read "Background Phases"() -> (w402:dbl[][][])
            n280 = node(w407, w412, "update_Axicon" ("function name"), w409, dbl[][] [[0.0, 0.0, 4.0], [0.0, 0.0, 0.0], [10.0, 0.0, 0.0]] ("Python Graph"), w411, w414, w415) -> (w406:refnum<k35>, w408:errorcluster, w401:dbl[][])  [unwired: 3 in, 2 out]
            n281 = Replace Array Subset(array=w402, new element=w401, index (dim 0)=2 ("index (page)")) -> (w404:dbl[][][])  [unwired: 2 in]
            n282 = local write "Background Phases"(w404) -> ()
          }
        }
        n283 = local read "Background Phases"() -> (w391:dbl[][][])
        n284 = local read "Control File Path"() -> (w392:path)
        n285 = local read "Aperture Mask"() -> (w378:sgl[][])
        n286 = node(w394, w392, "update_background" ("function name"), w393, dbl[][] [[0.0, 0.0, 4.0], [0.0, 0.0, 0.0], [10.0, 0.0, 0.0]] ("Python Graph"), w391, w378) -> (w381:errorcluster, w377:dbl[][])  [unwired: 2 in, 3 out]
        n287 = local write "Background  Graph"(w377) -> ()
      }
      event "Single Upload": Value Change {
        n288 = event-data() -> ()  [unwired: 1 in, 6 out]
        n289 = local read "Python session 2"() -> (w458:refnum<k35>)
        n290 = local read "Control File Path"() -> (w465:path)
        n291 = local read "Phases"() -> (w464:dbl[][][])
        n292 = node(w458, w465, "update_phase" ("function name"), w460, dbl[][] [[0.0, 0.0, 4.0], [0.0, 0.0, 0.0], [10.0, 0.0, 0.0]] ("Python Graph"), w464) -> (w459:errorcluster, →"Final Phase":dbl[][])  [unwired: 1 in, 3 out]
      }
      event "Start/Stop": Value Change {
        n293 = event-data() -> ()  [unwired: 1 in, 6 out]
        n294 = local read "Python session 2"() -> (w468:refnum<k35>)
        n295 = Close Python Session(session in=w468, error in=w467) -> (11:w466:errorcluster)
      }
    }
  }
  "slm error out 2" <- w12
  "Phases" <- w25
  "Control File Path" <- path "C:/Users/quantum/Desktop/SLM_GUI-SLM_GUI_ALL_Phases/SLM_GUI_Threaded_v3/slm_control.py" ("File Path")
  "Background Phases" <- w2
